vi "SMO.Transport.TestLauncher.vi"() -> (0 "error out":errorcluster)   [LabVIEW 2019, in "SMO.Transport.lvclass"]
uses:
  SMO.Transport.lvclass
  <vilib>/JKI/JKI SMO/SMO/Typedefs/SMOState --Enum.ctl
  C:/Program Files (x86)/National Instruments/LabVIEW 2019/vi.lib/JKI/JKI SMO/SMO/SMO.lvclass
  <vilib>/JKI/JKI SMO/SMO/SMO.lvclass/SMO.ctl
  <vilib>/JKI/JKI SMO/SMO/Private/ReftoDVR--SMO.vi
  <vilib>/JKI/JKI SMO/SMO/SMO.lvclass
panel:
  out "SMO State":T1
  # "Close Panel to stop the SMO\n(press the \"X\")"
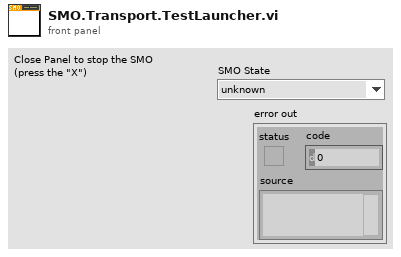
[diagram p1: front panel]
types:
  T1 = typedef "SMO.lvclass/SMOState --Enum.ctl" = enum16{"unknown", "Created", "Started", "Stopped"}
  T2 = typedef "SMO.lvclass/Public Events.ctl" = cluster{"Error":refnum<user-event>, "State":refnum<user-event>, "Reserve State":refnum<user-event>}
  T3 = cluster{"Event Registration Refnum":refnum<event-registration>}
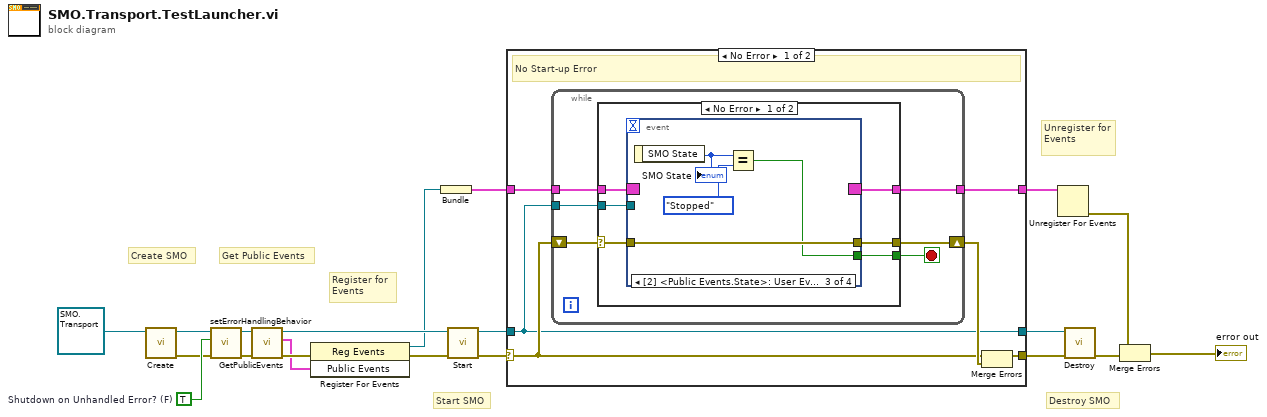
[diagram p0: block diagram]
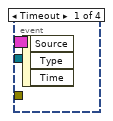
[diagram p2: hidden frame]
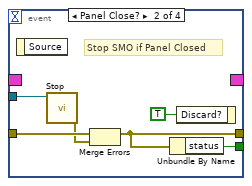
[diagram p3: hidden frame]
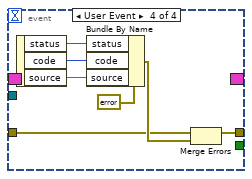
[diagram p4: hidden frame]
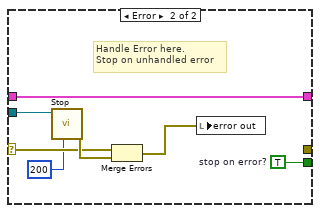
[diagram p5: hidden frame]
diagram:
  w16 = TRUE  # Shutdown on Unhandled Error? (F)
  # "Get Public Events"
  # "Start SMO"
  # "Destroy SMO"
  # "Create SMO"
  # "Unregister for Events"
  # "Register for Events"
  n1 = call <vilib>:"Create.vi"("SMO"=refnum<class "SMO.Transport.lvclass"> refnum ("SMO.Transport in")) -> ("error out"=w14:errorcluster, "SMO out"=w12:refnum<class "SMO.Transport.lvclass">)  [unwired: 8 in, 1 out]
  n2 = call <vilib>:"setErrorHandlingBehavior.vi"("error in (no error)"=w14, "Shutdown on Unhandled Error? (F)"=w16, "SMO in"=w12) -> ("error out"=w15:errorcluster, "SMO out"=w13:refnum<class "SMO.Transport.lvclass">)  [unwired: 7 in]
  n3 = call <vilib>:"GetPublicEvents.vi"("error in (no error)"=w15, "SMO"=w13) -> ("error out"=w10:errorcluster, "Public Events"=w9:T2, "SMO out"=w17:refnum<class "SMO.Transport.lvclass">)  [unwired: 7 in]
  n4 = register-events(error in=w10, w9) -> (reference out=w7:refnum<event-registration>, error out=w8:errorcluster)  [unwired: 1 in]
  n5 = Bundle("Event Registration Refnum"=w7) -> (w4:T3)  [unwired: 1 in]
  n6 = call <vilib>:"Start.vi"("error in (no error)"=w8, "SMO"=w17) -> ("error out"=w19:errorcluster, "SMO out"=w18:refnum<class "SMO.Transport.lvclass">)  [unwired: 8 in]
  n7 = case shown="No Error" w19 {
    selector: w19 -> [w22 w64]
    tunnel: [w26 w65] -> w3
    tunnel: w4 -> [w25 w65]
    tunnel: [w23 w64] -> w11
    tunnel: w18 -> [w21 w63]
    tunnel: [w21 w63] -> w20
    frame No Error {
      # "No Start-up Error"
      n8 = while {
        shift-right: [w31] -> w24
        shift-left: w22 -> [w27]
        tunnel: w25 -> [w30]
        tunnel: [w29] -> w26
        tunnel: w21 -> [w28]
        stop <- w32 stop-if-true
        n9 = case shown="No Error" w27 {
          selector: w27 -> [w33 w59]
          tunnel: [w38 w62] -> w32
          tunnel: [w37 _] -> w31
          tunnel: w30 -> [w36 w61]
          tunnel: [w35 w61] -> w29
          tunnel: w28 -> [w34 w58]
          frame No Error {
            n10 = event shown="[2] <Public Events.State>: User Event" {
              selector: w36 -> [_ _ _ _]
              dyn-events: [_ _ _ _] -> w35
              timeout: _ -> [_ _ _ _]
              tunnel: [_ w42 w45 _] -> w38
              tunnel: w34 -> [_ w44 _ _]
              tunnel: [_ w39 w46 w49] -> w37
              tunnel: w33 -> [_ w41 w46 w50]
              event Timeout {
                n11 = event-data() -> ()  [unwired: 1 in, 3 out]
              }
              event Panel Close? {
                # "Stop SMO if Panel Closed"
                n12 = event-data() -> ()  [unwired: 1 in, 1 out]
                n13 = call <vilib>:"Stop.vi"("SMO"=w44) -> ("error out"=w40:errorcluster)  [unwired: 9 in, 1 out]
                n14 = Merge Errors(w41, w40) -> (w39:errorcluster)
                n15 = Unbundle By Name(w39) -> ("status"=w42:bool)
                n16 = event-data("Discard?"=TRUE ("OK")) -> ()  [unwired: 1 in, 1 out]
              }
              event User Event {
                n17 = event-data() -> ("SMO State"=w48:T1)  [unwired: 1 in]
                "SMO State" <- w48
                n18 = Equal?(x=w48, y=SMOState_--Enum."Stopped") -> (x = y?=w45:bool)
              }
              event User Event {
                n19 = event-data() -> ("status"=w55:bool, "code"=w54:i32, "source"=w53:string)  [unwired: 1 in]
                n20 = Bundle By Name(cluster=errorcluster {"status"=FALSE, "code"=0, "source"=""} ("error out"), "status"=w55, "code"=w54, "source"=w53) -> (w51:errorcluster)
                n21 = Merge Errors(w50, w51) -> (w49:errorcluster)
              }
            }
          }
          frame Error {
            w62 = TRUE  # stop on error?
            # "Handle Error here.\nStop on unhandled error"
            n22 = call <vilib>:"Stop.vi"("timeout in ms (-1)"=200, "SMO"=w58) -> ("error out"=w60:errorcluster)  [unwired: 8 in, 1 out]
            n23 = Merge Errors(w59, w60) -> (w56:errorcluster)
            n24 = local write "error out"(w56) -> ()
          }
        }
      }
      n25 = Merge Errors(w22, w24) -> (w23:errorcluster)
    }
    frame Error {
      # "Error occured before starting the process"
    }
  }
  n26 = Unregister For Events(event registration refnum=w3) -> (error out=w5:errorcluster)  [unwired: 1 in]
  n27 = call <vilib>:"Destroy.vi"("error in (no error)"=w11, "SMO"=w20) -> ("error out"=w6:errorcluster)  [unwired: 9 in]
  n28 = Merge Errors(w5, w6) -> (→"error out":errorcluster)
